vi "test SSL Client HTTPS Request to Google.vi"(8 "error in (no error)":errorcluster, 11 "TestCase in":refnum<class "test SSL Client.lvclass">) -> (0 "error out":errorcluster, 3 "TestCase out":refnum<class "test SSL Client.lvclass">)   [LabVIEW 2013, in "test SSL Client.lvclass"]
uses:
  test SSL Client.lvclass
  NI OpenSSL Socket/SSL_Lib/SSL/SSL_Mode.ctl
  suite SSL Client/suite SSL Client/SSL Context.vi
  <vilib>/addons/_JKI Toolkits/VI Tester/TestCase.llb/TestCase.lvclass
  NI OpenSSL Socket/SSL_Lib/BIO/BIO.lvclass
  NI OpenSSL Socket/SSL_Lib/SSL-Context/SSL-Context.lvclass
  NI OpenSSL Socket/SSL_Lib/SSL/SSL.lvclass
  suite SSL Client/suite SSL Client/suite SSL Client.lvclass
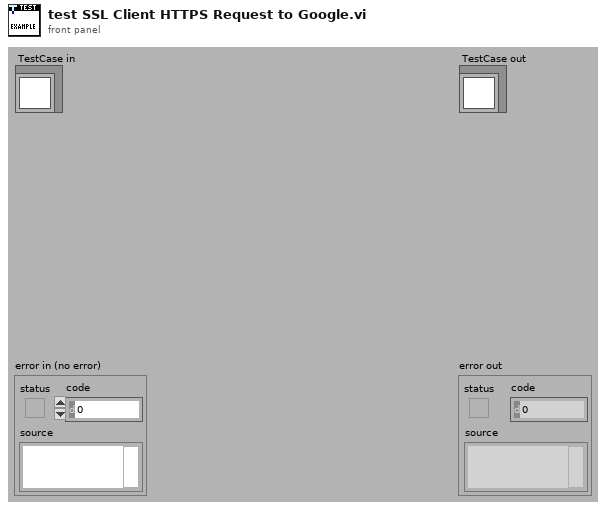
[diagram p1: front panel]
types:
  T1 = typedef "OpenSSL Socket.lvlib/SSL.lvclass/SSL_Mode.ctl" = i32
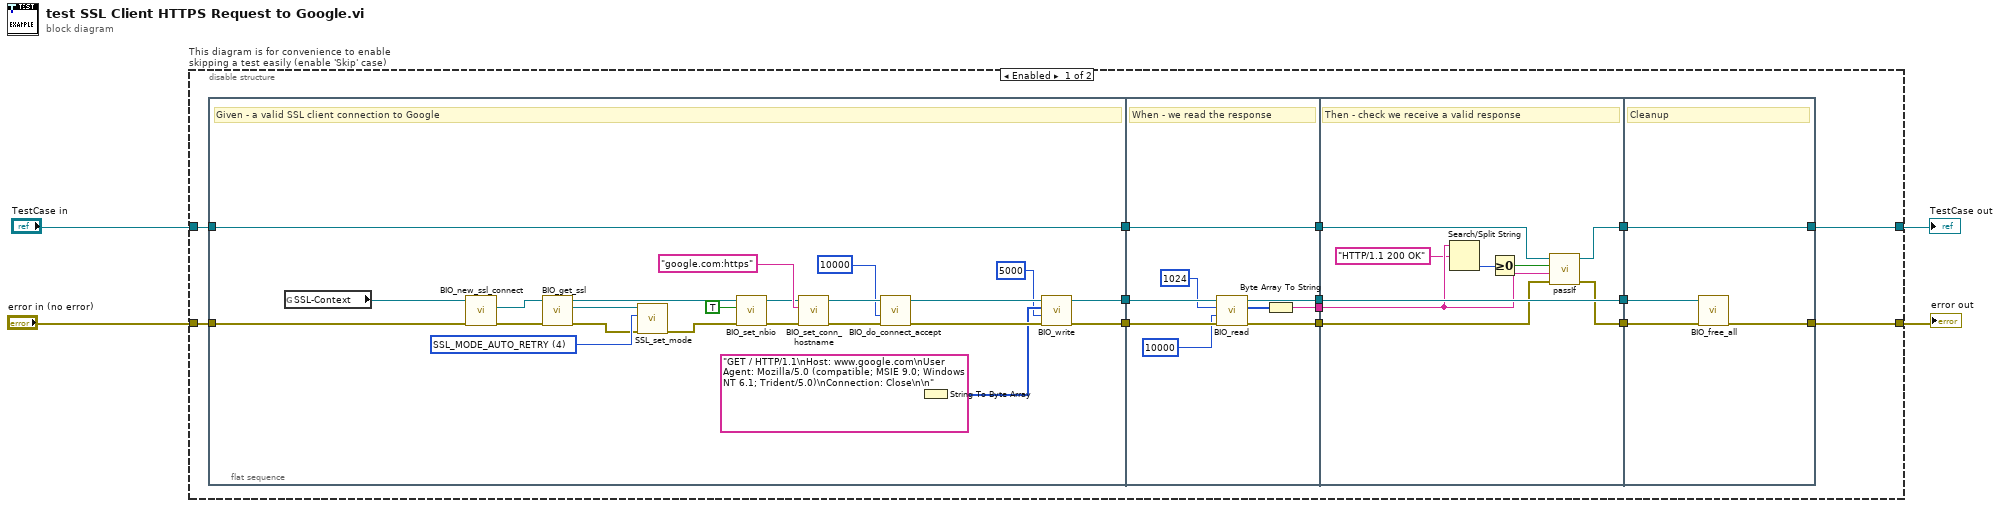
[diagram p0: block diagram]
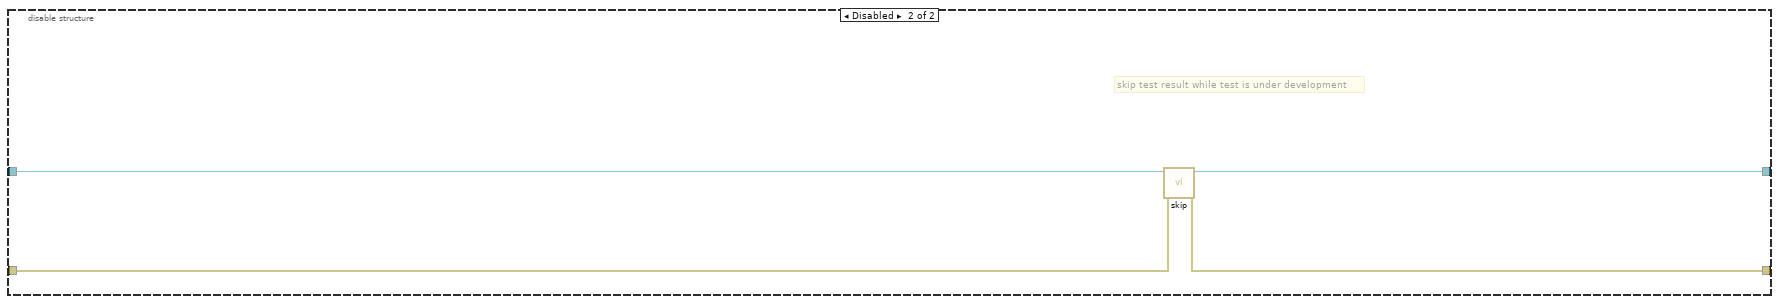
[diagram p2: hidden frame]
diagram:
  n1 = disable-structure "This diagram is for convenience to enable skipping a test easily (enable 'Skip' case)" shown="Enabled" {
    disable-tunnel: "TestCase in" -> [w12 w68]
    disable-tunnel: [w11 w66] -> w1
    disable-tunnel: [w10 w67] -> w3
    disable-tunnel: "error in (no error)" -> [w13 w65]
    frame Enabled {
      n2 = flat-sequence {
        tunnel: w13 -> [w29]
        tunnel: w12 -> [w38]
        tunnel: [w38] -> w18
        tunnel: [w37] -> w9
        tunnel: [w36] -> w8
        tunnel: [w51] -> w17
        tunnel: [w48] -> w16
        tunnel: w18 -> [w51]
        tunnel: w9 -> [w50]
        tunnel: w8 -> [w49]
        tunnel: [w44] -> w7
        tunnel: [w46] -> w6
        tunnel: [w56] -> w15
        tunnel: [w57] -> w14
        tunnel: w17 -> [w59]
        tunnel: w16 -> [w58]
        tunnel: w7 -> [w55]
        tunnel: w6 -> [w60]
        tunnel: [w60] -> w5
        tunnel: [w62] -> w10
        tunnel: [w64] -> w11
        tunnel: w15 -> [w64]
        tunnel: w14 -> [w63]
        tunnel: w5 -> [w61]
        frame #0 {
          w31 = T1 4 items=["None"=0, "SSL_MODE_ENABLE_PARTIAL_WRITE"=1, "SSL_MODE_ACCEPT_MOVING_WRITE_BUFFER"=2, "SSL_MODE_AUTO_RETRY"=4, "SSL_MODE_RELEASE_BUFFERS"=16, "SSL_MODE_SEND_FALLBACK_SCSV"=128] ("Mode")
          # "Given - a valid SSL client connection to Google"
          n3 = global read "SSL Context.vi" "SSL-Context"() -> (w28:refnum<class "SSL-Context.lvclass">)
          n4 = call "BIO_new_ssl_connect.vi"("error in (no error)"=w29, "SSL-Context in"=w28) -> ("error out"=w33:errorcluster, "BIO out"=w34:refnum<class "BIO.lvclass">)  [unwired: 7 in, 1 out]
          n5 = call "BIO_get_ssl.vi"("error in (no error)"=w33, "BIO in"=w34) -> ("error out"=w30:errorcluster, "SSL out"=w32:refnum<class "SSL.lvclass">, "BIO out"=w23:refnum<class "BIO.lvclass">)  [unwired: 7 in]
          n6 = call "SSL_set_mode.vi"("error in (no error)"=w30, "Mode"=w31, "SSL in"=w32) -> ("error out"=w26:errorcluster)  [unwired: 7 in, 1 out]
          n7 = call "BIO_set_nbio.vi"("error in (no error)"=w26, "Non-Blocking?"=TRUE, "BIO in"=w23) -> ("error out"=w24:errorcluster, "BIO out"=w25:refnum<class "BIO.lvclass">)  [unwired: 7 in]
          n8 = call "BIO_set_conn_hostname.vi"("error in (no error)"=w24, "Hostname"="google.com:https", "BIO in"=w25) -> ("error out"=w41:errorcluster, "BIO out"=w35:refnum<class "BIO.lvclass">)  [unwired: 7 in]
          n9 = call "BIO_do_connect_accept.vi"("error in (no error)"=w41, "Timeout (10000ms)"=u32 10000, "BIO in"=w35) -> ("error out"=w40:errorcluster, "BIO out"=w39:refnum<class "BIO.lvclass">)  [unwired: 7 in]
          n10 = String To Byte Array(string="GET / HTTP/1.1\nHost: www.google.com\nUser Agent: Mozilla/5.0 (compatible; MSIE 9.0; Windows NT 6.1; Trident/5.0)\nConnection: Close\n\n" ("String to write")) -> (unsigned byte array=w21:u8[])
          n11 = call "BIO_write.vi"("error in (no error)"=w40, "Timeout (10000ms)"=u32 5000, "Bytes to write"=w21, "BIO in"=w39) -> ("error out"=w37:errorcluster, "BIO out"=w36:refnum<class "BIO.lvclass">)  [unwired: 5 in, 1 out]
        }
        frame #1 {
          # "When - we read the response"
          n12 = call "BIO_read.vi"("error in (no error)"=w50, "Timeout (10000ms)"=u32 10000, "bytes to read"=1024, "BIO in"=w49) -> ("error out"=w48:errorcluster, "Bytes read"=w47:u8[], "BIO out"=w46:refnum<class "BIO.lvclass">)  [unwired: 5 in]
          n13 = Byte Array To String(unsigned byte array=w47) -> (string=w44:string)
        }
        frame #2 {
          # "Then - check we receive a valid response"
          n14 = Search/Split String(string=w55, search string/char (-)="HTTP/1.1 200 OK" ("regular expression")) -> (offset of match=w53:i32)  [unwired: 1 in, 2 out]
          n15 = Greater Or Equal To 0?(x=w53) -> (x >= 0?=w52:bool)
          n16 = call-dynamic "passIf.vi"("error in (no error)"=w58, "message (\"\")"=w55, "pass"=w52, "TestCase in"=w59) -> ("error out"=w57:errorcluster, "TestCase out"=w56:refnum<class "test SSL Client.lvclass">)  [unwired: 6 in]
        }
        frame #3 {
          # "Cleanup"
          n17 = call "BIO_free_all.vi"("error in (no error)"=w63, "BIO in"=w61) -> ("error out"=w62:errorcluster)  [unwired: 9 in]
        }
      }
    }
    frame Disabled {
      # "skip test result while test is under development"
      n18 = call <vilib>:"skip.vi"("error in (no error)"=w65, "TestCase in"=w68) -> ("error out"=w67:errorcluster, "TestCase out"=w66:refnum<class "test SSL Client.lvclass">)  [unwired: 8 in]
    }
  }
  "error out" <- w3
  "TestCase out" <- w1
